vi "push array double.vi"(0 "Array":dbl[](array[numeric]), 2 "mode":enum16{"forwards (i=0)", "backwards (i=n)"}(ring), 11 "Element":dbl) -> (8 "Array out":dbl[](array[numeric]))   [LabVIEW 2010, in "Licor-Steuerung.lvlib"]
uses:
  Licor-Steuerung.lvlib
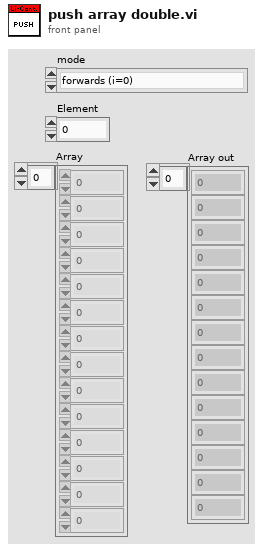
[diagram p1: front panel]
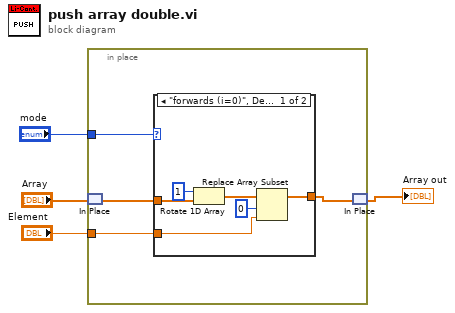
[diagram p0: block diagram]
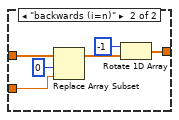
[diagram p2: hidden frame]
diagram:
  n1 = in-place {
    in-place-border: "mode" -> [w8]
    in-place-border: "Element" -> [w7]
    n2 = in-place-match #1("Array") -> (w6:dbl[])
    n3 = case shown="\"forwards (i=0)\", Default" w8 {
      tunnel: w6 -> [w14 w19]
      tunnel: w7 -> [w11 w18]
      tunnel: [w9 w15] -> w5
      frame "forwards (i=0)", Default {
        n4 = Rotate 1D Array(1:w14, 2:1 ("n")) -> (0:w12:dbl[])
        n5 = Replace Array Subset(array=w12, new element=w11, index=0 ("Index")) -> (w9:dbl[])
      }
      frame "backwards (i=n)" {
        n6 = Replace Array Subset(array=w19, new element=w18, index=0 ("Index")) -> (w16:dbl[])
        n7 = Rotate 1D Array(1:w16, 2:-1 ("n")) -> (0:w15:dbl[])
      }
    }
    n8 = in-place-match #1(w5) -> (→"Array out":dbl[])
  }
